vi "Configure Front Panel Layout.vi"   [LabVIEW 2012]
uses:
  vi.lib/Front Panel Layout/Configure Front Panel Layout/NI_SE_Config Front Panel Layout.lvlib
types:
  T1 = enum32{"Invalid", "Standard", "Closed", "Hidden", "Minimized", "Maximized"}
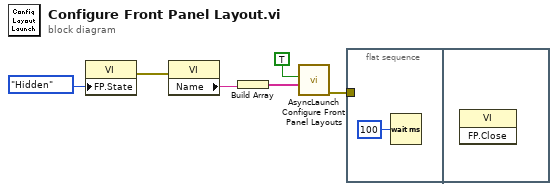
[diagram p0: block diagram]
diagram:
  n1 = property class="VI"("FP.State"=T1."Hidden" ("Front Panel Window:State")) -> (error out=w1:errorcluster)  [unwired: 2 in, 1 out]
  n2 = property class="VI"(error in=w1) -> ("Name"=w6:string)  [unwired: 1 in, 2 out]
  n3 = Build Array(w6) -> (w3:string[])
  n4 = call "AsyncLaunch Configure Front Panel Layouts.vi"("VIs to exclude"=w3, "close window when done? (F)"=TRUE) -> ("error out"=w2:errorcluster)  [unwired: 9 in]
  n5 = flat-sequence {
    tunnel: w2 -> [_]
    frame #0 {
      n6 = Wait (ms)(milliseconds to wait=u32 100) -> ()  [unwired: 1 out]
    }
    frame #1 {
      n7 = invoke class="VI" method="FP.Close"() -> ()  [unwired: 3 in, 3 out]
    }
  }
